vi "niRFUtil MEAS Waveform Statistics (complex wfm).vi"(2 "Waveform In":T1 {"y" format="%.2f"; "dx" format="%^.2e"; "x0" format="%^.2e"}) -> (5 "Start":dbl format="%^.2e", 6 "Interval":dbl format="%^.2e", 7 "End + Interval":dbl format="%^.2e", 8 "Duration":dbl format="%^.2e")   [LabVIEW 2015, in "niRFUtil.lvlib"]
doc: "(c) Copyright 2006, National Instruments, Inc. This VI may not be duplicated, sold, or distributed without written consent from National Instruments."
uses:
  niRFUtil.lvlib
  Includes/niRFUtil INC Complex Waveform.ctl
  Includes/niRFUtil INC Complex Array.ctl
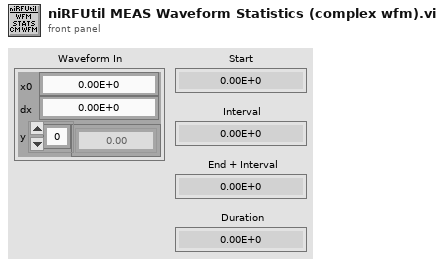
[diagram p1: front panel]
types:
  T1 = typedef "niRFUtil.lvlib/niRFUtil INC Complex Waveform.ctl" = cluster{"x0":dbl, "dx":dbl, "y":T2}
  T2 = typedef "niRFUtil.lvlib/niRFUtil INC Complex Array.ctl" = csg[]
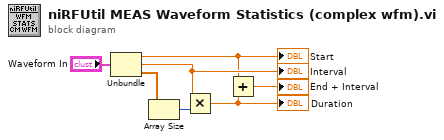
[diagram p0: block diagram]
diagram:
  n1 = Unbundle("Waveform In") -> ("x0"=w3:dbl, "dx"=w5:dbl, "y"=w6:T2)
  "Start" <- w3
  "Interval" <- w5
  n2 = Array Size(array=w6) -> (size(s)=w2:i32)
  n3 = Multiply(x=w5, y=w2) -> (x*y=w1:dbl)
  "Duration" <- w1
  n4 = Add(x=w3, y=w1) -> (x+y=→"End + Interval":dbl)
